vi "LEP_RV_GetWordsOfALine.vi"(8 "error out":errorcluster, 11 "Initial String":string) -> (0 "error IO":errorcluster, 3 "Array containing the words (tokens) of a string":string[](array[string]))   [LabVIEW 2011]
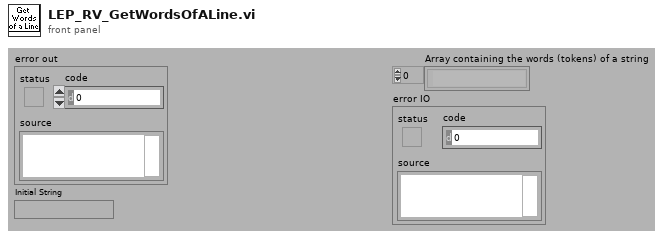
[diagram p1: front panel]
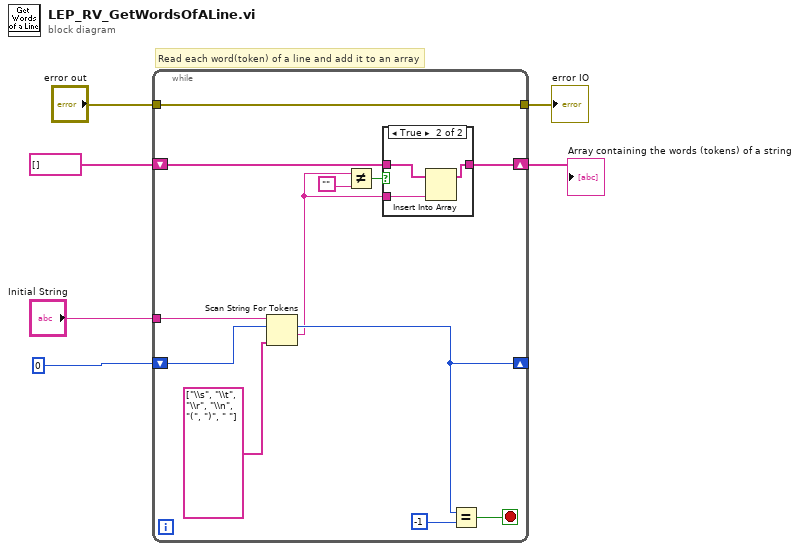
[diagram p0: block diagram]
diagram:
  # "Read each word(token) of a line and add it to an array"
  n1 = while {
    tunnel: "error out" -> [w15]
    tunnel: [w15] -> w3
    tunnel: "Initial String" -> [w16]
    shift-right: [w13] -> w2
    shift-left: string[] [] -> [w14]
    shift-right: [w11] -> _
    shift-left: 0 ("offset past token") -> [w12]
    stop <- w18 stop-if-true
    n2 = Scan String For Tokens(6:string[] ["\\s", "\\t", "\\r", "\\n", "(", ")", " "] ("delimiters (\\s,\\t,\\r,\\n)"), 8:w12, 9:w16) -> (1:w10:string, 2:w11:i32)  [unwired: 3 in, 2 out]
    n3 = Not Equal?(x=w10, y="") -> (x != y?=w8:bool)
    n4 = case shown="True" w8 {
      tunnel: w14 -> [w19 w22]
      tunnel: w10 -> [_ w21]
      tunnel: [w19 w20] -> w13
      frame False {
      }
      frame True {
        n5 = Insert Into Array(array=w22, new element=w21) -> (w20:string[])  [unwired: 1 in]
      }
    }
    n6 = Equal?(x=w11, y=-1) -> (x = y?=w18:bool)
  }
  "Array containing the words (tokens) of a string" <- w2
  "error IO" <- w3
